vi "CommandSendCvtr.vi"(10 "Para":u8, 11 "Cmd":string="LWHEEL") -> (2 "连接的字符串":string)   [LabVIEW 2012, in "User_define.lvlib"]
uses:
  User_define.lvlib
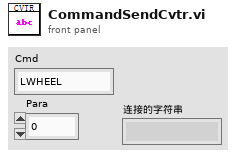
[diagram p1: front panel]
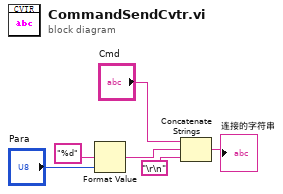
[diagram p0: block diagram]
diagram:
  n1 = Format Value ("格式化值")(format string="%d" ("格式字符串"), value (0)="Para") -> (output string=w2:string)  [unwired: 1 in]
  n2 = Concatenate Strings("Cmd", w2, "\r\n") -> (→"连接的字符串":string)
